vi "Trial Based Experiment Runner.vi"() -> ()   [LabVIEW 2012]
doc: "Use this template to measure or generate signals using the DAQ Assistant Express VI and NI-DAQmx. Double click the DAQ Assistant Express VI to launch a configuration wizard which steps you through configuring a measurement or generation.\n\nNote: You must have an NI-DAQmx compatible device installed to use this Express VI. Refer to the DAQ Quick Start Guide for NI-DAQ 7.0 for a list of compatible devices."
uses:
  Trial Based Experiment.lvsc/State.ctl
  Acquisition/BehaviorData/BehaviorData.lvclass
  <vilib>/Utility/error.llb/DialogType.ctl
  Experiments/EyeCalibration/EyeCalibration.lvclass
  Experiments/ClassDiscrimination/ClassDiscrimination.lvclass
  Experiments/FlePhysEffExperiment/FlePhysEffExperiment.lvclass
  Experiments/MultDimExperiment/MultDimExperiment.lvclass
  Experiments/DotMappingExperiment/DotMappingExperiment.lvclass
  Experiments/FlashLagExperiment/FlashLagExperiment.lvclass
  Experiments/FleTraining/FleTraining.lvclass
  Experiments/OriDiscExperiment/OriDiscExperiment.lvclass
  Experiments/MoviesExperiment/MoviesExperiment.lvclass
  Experiments/MouseMultiDim/MouseMultiDim.lvclass
  Experiments/WNOriDiscExperiment/WNOriDiscExperiment.lvclass
  Experiments/MouseBar/MouseBar.lvclass
  Experiments/MouseDotMapping/MouseDotMapping.lvclass
  Experiments/WhiteNoiseOrientationDetection/WhiteNoiseOrientationDetection.lvclass
  MatlabExperiment/MatlabExperiment.lvclass
  Trial Based Experiment.lvsc/Trigger.ctl
  Trial Based Experiment.lvsc/Inputs.ctl
  TrialBasedExperiment.lvclass
  <vilib>/Statechart/Common/IntGuid.ctl
  <vilib>/Statechart/Common/DbgID.ctl
  Trial Based Experiment.lvsc/StatechartState.ctl
  Trial Based Experiment.lvsc/CompanionDiagram.vi/162/SC Main.vi
  <vilib>/Statechart/Infrastructure/RTStatechart/RunTime SCN.xnode
  Trial Based Experiment.lvsc/Outputs.ctl
  Trial Based Experiment.lvsc
  Core SubVIs/Core SubVIs.lvlib
  <vilib>/Statechart/Common/NI_SC_LVSCCommonFiles.lvlib
panel:
  out "Stopped":bool
  in  "Emergency Stop":bool
  out "Data Process Loop":i32
  out "Data Acquire Loop":i32
  out "error out":errorcluster
  out "State":T1
  in  "Experiment":T2(ring)
  out "Missed Updates":dbl
  out "Fixated":bool
  in  "Squirt Time(ms)":u32=50
  in  "Pause":bool
  out "Terminated?":bool
  in  "Stop":bool
  in  "Juice":bool
  # "TODO:\n1. Make EyeParams me properly set\n2. Synchronization"
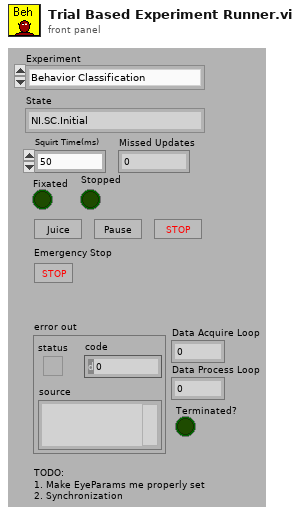
[diagram p1: front panel]
types:
  T1 = typedef "Trial Based Experiment.lvsc/State.ctl" = enum16{"NI.SC.Initial", "NI.SC.History", "NI.SC.ShallowHistory", "NI.SC.Terminal", "Cleanup", "State", "State\\Region\\Pause", "State\\Region\\Response Period", "State\\Region\\Delay Period", "State\\Region\\Hold Fixation", "State\\Region\\Acquire Fixation", "State\\Region\\Abort Trial", "State\\Region\\End Trial", "State\\Region\\Intertrial", "State\\Region\\Start Trial"}
  T2 = enum16{"Behavior Classification", "DotMappingExperiment", "Eye Calibration", "FlePhysEffExperiment", "MultDimExperiment", "FlashLagExperiment", "FleTraining", "OriDiscExperiment", "WNOriDetectExperiment", "WNOriDiscExperiment", "MovieExperiment", "MouseMultiDim", "MouseDotMapping", "MouseBarExperiment"}
  T3 = typedef "DialogType.ctl" = u16
  T4 = typedef "StimulationPrimary.ctl" = cluster{"setup":u8, "subject_id":i32, "session_start_time":dbl, "stim_start_time":dbl}
  T5 = typedef "Trial Based Experiment.lvsc/Inputs.ctl" = cluster{"Timing":cluster{"Intertrial time":dbl, "Acquire fixation time":dbl, "Hold fixation time":dbl, "Delay period time":dbl, "Response time":dbl, "Reward":dbl, "Punish time":dbl}, "Stop":bool, "Control states":cluster{"Fixated":bool, "Centered":bool}, "Pause":bool, "Hammer running":bool, "Experiment":refnum<class "TrialBasedExperiment.lvclass">, "error in":errorcluster}
  T6 = typedef "Trial Based Experiment.lvsc/Trigger.ctl" = enum16{"NULL", "Fixated", "Broke Fixation", "Stop", "Correct Response", "Incorrect Response", "Timeout"}
  T7 = enum16{"Get Time", "Get Elapsed Time", "Reset Elapsed Time"}
  T8 = typedef "NI_SC_LVSCCommonFiles.lvlib/IntGuid.ctl" = cluster{"Data1":u32, "Data2":u16, "Data3":u16, "Data4":u8, "Data5":u8, "Data6":u8, "Data11":u8, "Data9":u8, "Data10":u8, "Data8":u8, "Data7":u8}
  T9 = typedef "NI_SC_LVSCCommonFiles.lvlib/DbgID.ctl" = cluster{"VIRef":u32, "IntGUID":T8}
  T10 = typedef "Trial Based Experiment.lvsc/Outputs.ctl" = cluster{"Experiment":refnum<class "TrialBasedExperiment.lvclass">, "Timeout":dbl, "error out":errorcluster}
  T11 = typedef "Trial Based Experiment.lvsc/StatechartState.ctl" = T1[]
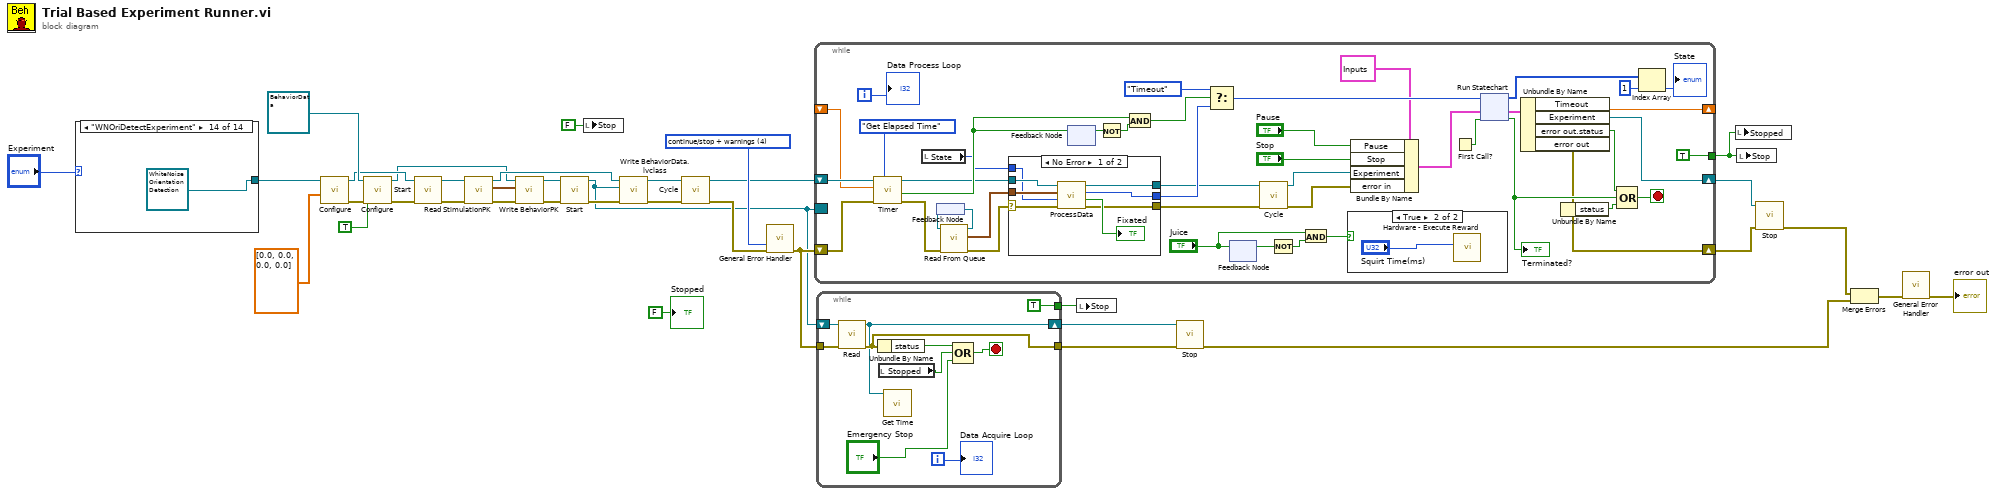
[diagram p0: block diagram]
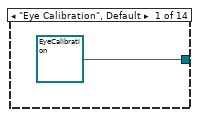
[diagram p2: hidden frame]
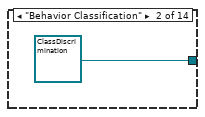
[diagram p3: hidden frame]
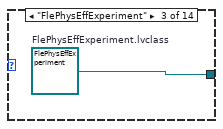
[diagram p4: hidden frame]
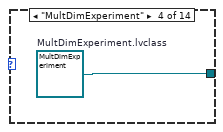
[diagram p5: hidden frame]
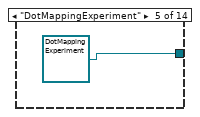
[diagram p6: hidden frame]
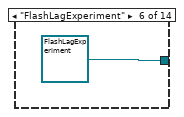
[diagram p7: hidden frame]
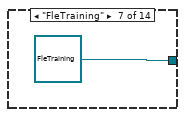
[diagram p8: hidden frame]
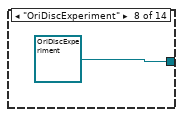
[diagram p9: hidden frame]
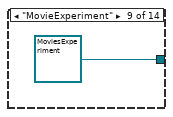
[diagram p10: hidden frame]
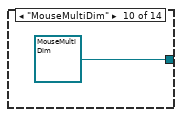
[diagram p11: hidden frame]
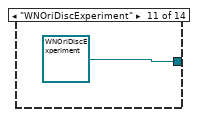
[diagram p12: hidden frame]
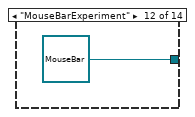
[diagram p13: hidden frame]
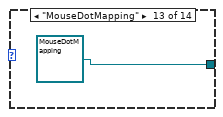
[diagram p14: hidden frame]
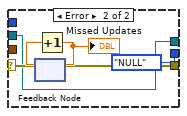
[diagram p15: hidden frame]
diagram:
  w35 = T3 4 items=["no dialog", "OK message", "continue or stop message", "OK message + warnings", "continue/stop + warnings"] ("type of dialog (OK msg:1)")
  n1 = case shown="\"WNOriDetectExperiment\"" "Experiment" {
    tunnel: [refnum<class "EyeCalibration.lvclass"> refnum ("EyeCalibration.lvclass") refnum<class "ClassDiscrimination.lvclass"> refnum ("ClassDiscrimination.lvclass") w39 w40 refnum<class "DotMappingExperiment.lvclass"> refnum ("DotMappingExperiment.lvclass") refnum<class "FlashLagExperiment.lvclass"> refnum ("FlashLagExperiment.lvclass") refnum<class "FleTraining.lvclass"> refnum ("FleTraining.lvclass") refnum<class "OriDiscExperiment.lvclass"> refnum ("OriDiscExperiment.lvclass") refnum<class "MoviesExperiment.lvclass"> refnum ("MoviesExperiment.lvclass") refnum<class "MouseMultiDim.lvclass"> refnum ("MouseMultiDim.lvclass") refnum<class "WNOriDiscExperiment.lvclass"> refnum ("WNOriDiscExperiment.lvclass") refnum<class "MouseBar.lvclass"> refnum ("MouseBar.lvclass") refnum<class "MouseDotMapping.lvclass"> refnum ("MouseDotMapping.lvclass") refnum<class "WhiteNoiseOrientationDetection.lvclass"> refnum ("WhiteNoiseOrientationDetection.lvclass")] -> w29
    frame "Eye Calibration", Default {
    }
    frame "Behavior Classification" {
    }
    frame "FlePhysEffExperiment" {
      w39 = refnum<class "FlePhysEffExperiment.lvclass"> refnum  # FlePhysEffExperiment.lvclass
    }
    frame "MultDimExperiment" {
      w40 = refnum<class "MultDimExperiment.lvclass"> refnum  # MultDimExperiment.lvclass
    }
    frame "DotMappingExperiment" {
    }
    frame "FlashLagExperiment" {
    }
    frame "FleTraining" {
    }
    frame "OriDiscExperiment" {
    }
    frame "MovieExperiment" {
    }
    frame "MouseMultiDim" {
    }
    frame "WNOriDiscExperiment" {
    }
    frame "MouseBarExperiment" {
    }
    frame "MouseDotMapping" {
    }
    frame "WNOriDetectExperiment" {
    }
  }
  n2 = call-dynamic "Configure.vi"("Eye Params"=dbl[] [0.0, 0.0, 0.0, 0.0] ("Init Eye Params"), "TrialBasedExperiment in"=w29) -> ("error out"=w25:errorcluster, "TrialBasedExperiment out"=w24:refnum<class "MatlabExperiment.lvclass">)  [unwired: 8 in]
  n3 = call-dynamic "Configure.vi"("error in (no error)"=w25, "Record"=TRUE, "BehaviorData in"=refnum<class "BehaviorData.lvclass"> refnum ("BehaviorData.lvclass")) -> ("error out"=w16:errorcluster, "BehaviorData out"=w11:refnum<class "BehaviorData.lvclass">)  [unwired: 7 in]
  n4 = call-dynamic "Start.vi"("error in (no error)"=w16, "TrialBasedExperiment in"=w24) -> ("error out"=w17:errorcluster, "TrialBasedExperiment out"=w18:refnum<class "MatlabExperiment.lvclass">)  [unwired: 8 in]
  n5 = call-dynamic "Read StimulationPK.vi"("error in (no error)"=w17, "TrialBasedExperiment in"=w18) -> ("error out"=w8:errorcluster, "StimulationPK"=w12:T4, "TrialBasedExperiment out"=w15:refnum<class "MatlabExperiment.lvclass">)  [unwired: 7 in]
  n6 = call-dynamic "Write BehaviorPK.vi"("error in (no error)"=w8, "BehaviorPK"=w12, "BehaviorData in"=w11) -> ("error out"=w9:errorcluster, "BehaviorData out"=w10:refnum<class "BehaviorData.lvclass">)  [unwired: 7 in]
  n7 = call-dynamic "Start.vi"("error in (no error)"=w9, "Electrophysiology in"=w10) -> ("error out"=w23:errorcluster, "Electrophysiology out"=w13:refnum<class "BehaviorData.lvclass">)  [unwired: 8 in]
  n8 = local write "Stop"(FALSE ("Stop")) -> ()
  n9 = call-dynamic "Write BehaviorData.lvclass.vi"("error in (no error)"=w23, "BehaviorData.lvclass"=w13, "TrialBasedExperiment in"=w15) -> ("error out"=w22:errorcluster, "TrialBasedExperiment out"=w21:refnum<class "MatlabExperiment.lvclass">)  [unwired: 7 in]
  n10 = call-dynamic "Cycle.vi"("error in (no error)"=w22, "MatlabExperiment In"=w21) -> ("error out"=w33:errorcluster, "MatlabExperiment Out"=w34:refnum<class "MatlabExperiment.lvclass">)  [unwired: 8 in]
  n11 = call <vilib>:"General Error Handler.vi"("type of dialog (OK msg:1)"=w35, "error in (no error)"=w33) -> ("error out"=w14:errorcluster)  [unwired: 9 in, 4 out]
  n12 = while {
    shift-right: [w84] -> w31
    shift-left: w34 -> [w61]
    shift-right: [w81] -> _
    shift-left: _ -> [w59]
    tunnel: [TRUE] -> w1
    shift-right: [w63] -> w30
    shift-left: w14 -> [w53]
    border: w13 -> [_]
    i -> [w54]
    stop <- w76 stop-if-true
    n13 = call-dynamic "Timer.vi"("Method"=T7."Get Elapsed Time", "error in (no error)"=w53, "Timeout"=w59, "BehaviorData in"=w61) -> ("error out"=w52:errorcluster, "Timeout"=w58:bool, "BehaviorData out"=w55:refnum<class "TrialBasedExperiment.lvclass">)  [unwired: 4 in, 1 out]
    n14 = local read "State"() -> (w51:T1)
    n15 = feedback #1() -> (w56:refnum<class "BehaviorData.lvclass">)
    n16 = call-dynamic "Read From Queue.vi"("error in (no error)"=w52, "BehaviorData in"=w56) -> ("error out"=w66:errorcluster, "Array"=w67:waveform(dbl)[], "BehaviorData out"=w57:refnum<class "BehaviorData.lvclass">)  [unwired: 7 in]
    n17 = feedback-in #1(w57) -> ()
    n18 = case shown="No Error" w66 {
      selector: w66 -> [w101 w105]
      tunnel: [w100 w105] -> w64
      tunnel: w67 -> [w99 _]
      tunnel: [w98 Trigger."NULL" ("Trigger")] -> w82
      tunnel: w55 -> [w97 w103]
      tunnel: [w96 w103] -> w65
      tunnel: w51 -> [w95 _]
      frame No Error {
        n19 = call-dynamic "ProcessData.vi"("error in (no error)"=w101, "State"=w95, "Analog Data"=w99, "TrialBasedExperiment in"=w97) -> ("error out"=w100:errorcluster, "Fixated"=→"Fixated":bool, "Trigger"=w98:T6, "TrialBasedExperiment out"=w96:refnum<class "TrialBasedExperiment.lvclass">)  [unwired: 4 in]
      }
      frame Error {
        n20 = feedback #2() -> (w106:dbl)  [unwired: 1 in]
        n21 = Increment(x=w106) -> (x+1=w107:dbl)
        "Missed Updates" <- w107
        n22 = feedback-in #2(w107) -> ()
      }
    }
    n23 = feedback #3() -> (w90:bool)  [unwired: 1 in]
    n24 = feedback-in #3(w58) -> ()
    n25 = Not(x=w90) -> (.not. x?=w89:bool)
    n26 = And(x=w58, y=w89) -> (x .and. y?=w80:bool)
    n27 = Select(t=Trigger."Timeout" ("Trigger"), s=w80, f=w82) -> (s? t:f=w74:T6)
    n28 = feedback #4() -> (w88:bool)  [unwired: 1 in]
    n29 = feedback-in #4("Juice") -> ()
    n30 = call-dynamic "Cycle.vi"("error in (no error)"=w64, "TrialBasedExperiment In"=w65) -> ("error out"=w75:errorcluster, "TrialBasedExperiment Out"=w79:refnum<class "TrialBasedExperiment.lvclass">)  [unwired: 8 in]
    n31 = Not(x=w88) -> (.not. x?=w87:bool)
    n32 = And(x="Juice", y=w87) -> (x .and. y?=w85:bool)
    n33 = case shown="True" w85 {
      frame False {
      }
      frame True {
        n34 = call "Hardware - Execute Reward.vi"("Reward Time (200 ms)"="Squirt Time(ms)") -> ()  [unwired: 1 in, 10 out]
      }
    }
    n35 = Bundle By Name(cluster=T5 {"Timing"={"Intertrial time"=0.0, "Acquire fixation time"=0.0, "Hold fixation time"=0.0, "Delay period time"=0.0, "Response time"=0.0, "Reward"=0.0, "Punish time"=0.0}, "Stop"=FALSE, "Control states"={"Fixated"=FALSE, "Centered"=FALSE}, "Pause"=FALSE, "Hammer running"=FALSE, "Experiment"=refnum, "error in"={"status"=FALSE, "code"=0, "source"=""}} ("Inputs"), "Pause"="Pause", "Stop"="Stop", "Experiment"=w79, "error in"=w75) -> (w73:T5)
    n36 = First Call?() -> (First Call?: T/F=w92:bool)
    n37 = xnode "Run Statechart"("Init?"=w92, "Inputs"=w73, "Trigger"=w74) -> ("Terminated?"=w77:bool, "Outputs"=w91:T10, "Active States"=w72:T11)
    "Terminated?" <- w77
    n38 = Unbundle By Name(w91) -> ("Timeout"=w81:dbl, "Experiment"=w84:refnum<class "TrialBasedExperiment.lvclass">, "error out.status"=w78:bool, "error out"=w63:errorcluster)
    n39 = Unbundle By Name(w63) -> ("status"=w62:bool)
    n40 = Compound Arithmetic op=OR(w78, w77, w62) -> (w76:bool)
    n41 = Index Array(array=w72, index=1) -> (element=→"State":T1)
    "Data Process Loop" <- w54
  }
  n42 = while {
    tunnel: [w205] -> w7
    tunnel: w14 -> [w204]
    shift-right: [w201] -> w6
    shift-left: w13 -> [w208]
    tunnel: [TRUE] -> w28
    i -> [w203]
    stop <- w206 stop-if-true
    n43 = call-dynamic "Read.vi"("error in (no error)"=w204, "Behavior in"=w208) -> ("error out"=w205:errorcluster, "Behavior out"=w201:refnum<class "BehaviorData.lvclass">)  [unwired: 8 in]
    n44 = Unbundle By Name(w205) -> ("status"=w207:bool)
    n45 = local read "Stopped"() -> (w199:bool)
    n46 = call-dynamic "Get Time.vi"("BehaviorData in"=w201) -> ()  [unwired: 8 in, 3 out]
    n47 = Compound Arithmetic op=OR(w207, w199, "Emergency Stop") -> (w206:bool)
    "Data Acquire Loop" <- w203
  }
  n48 = local write "Stop"(w28) -> ()
  n49 = call-dynamic "Stop.vi"("error in (no error)"=w7, "Electrophysiology in"=w6) -> ("error out"=w5:errorcluster)  [unwired: 8 in, 1 out]
  n50 = local write "Stopped"(w1) -> ()
  n51 = local write "Stop"(w1) -> ()
  n52 = call-dynamic "Stop.vi"("error in (no error)"=w30, "TrialBasedExperiment in"=w31) -> ("error out"=w4:errorcluster)  [unwired: 8 in, 1 out]
  n53 = Merge Errors(w4, w5) -> (w3:errorcluster)
  n54 = call <vilib>:"General Error Handler.vi"("error in (no error)"=w3) -> ("error out"=→"error out":errorcluster)  [unwired: 10 in, 4 out]
  "Stopped" <- FALSE ("Stopped")
